vi "HCC Build Save Data Array.vi"(10 "Washer Array":T1[](array[typedef])) -> (2 "appended array":string[](array[string]))   [LabVIEW 2011]
uses:
  HCC Data.ctl
  Washer Status Ctrl.ctl
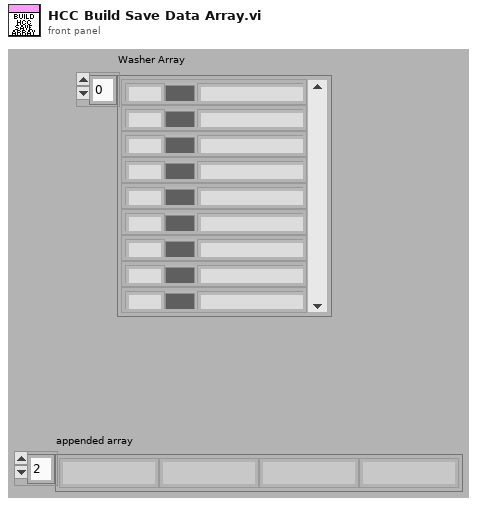
[diagram p1: front panel]
types:
  T1 = typedef "HCC Data.ctl" = cluster{"Station":string, "Color":u32, "Status":T2, "Error Time":string, "Com Err Count":u32, "Debug Log":string}
  T2 = typedef "Washer Status Ctrl.ctl" = enum16{"Running", "Err", "No Com", "No Conf"}
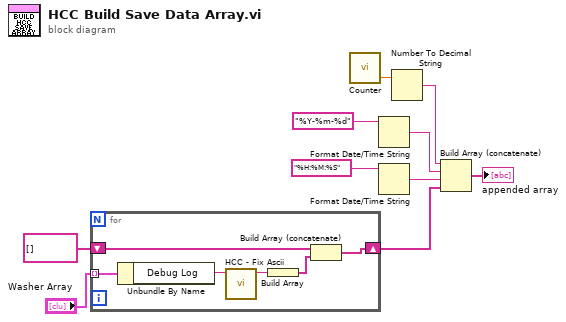
[diagram p0: block diagram]
diagram:
  n1 = for {
    tunnel: "Washer Array" -> [w16] mode=indexing
    shift-right: [w15] -> w8
    shift-left: string[] [] -> [w14]
    n2 = Unbundle By Name(w16) -> ("Debug Log"=w13:string)
    n3 = call "HCC - Fix Ascii.vi"("input string"=w13) -> ("result string"=w12:string)  [unwired: 10 in]
    n4 = Build Array(w12) -> (w11:string[])
    n5 = Build Array (concatenate)(w14, w11) -> (w15:string[])
  }
  n6 = call "Counter.vi"() -> ("Count"=w10:dbl)  [unwired: 11 in]
  n7 = Format Date/Time String(time format string (%c)="%Y-%m-%d") -> (date/time string=w5:string)  [unwired: 2 out]
  n8 = Format Date/Time String(time format string (%c)="%H:%M:%S") -> (date/time string=w3:string)  [unwired: 2 out]
  n9 = Number To Decimal String(number=w10) -> (decimal integer string=w7:string)  [unwired: 1 in]
  n10 = Build Array (concatenate)(w7, w5, w3, w8) -> (→"appended array":string[])
